vi "QueueDriver.vi"(0 "Queue Name":string, 5 "State":string, 7 "Array of States":string[](array[string]), 11 "error in (no error)":errorcluster, 13 "Operations":T1) -> (4 "Dequeued State":string, 15 "error out":errorcluster)   [LabVIEW 2020]
doc: "QueueDriver.vi is the SubVI which handles the states that is going to be operated in the Main VI."
uses:
  Typedefs/Operations.ctl
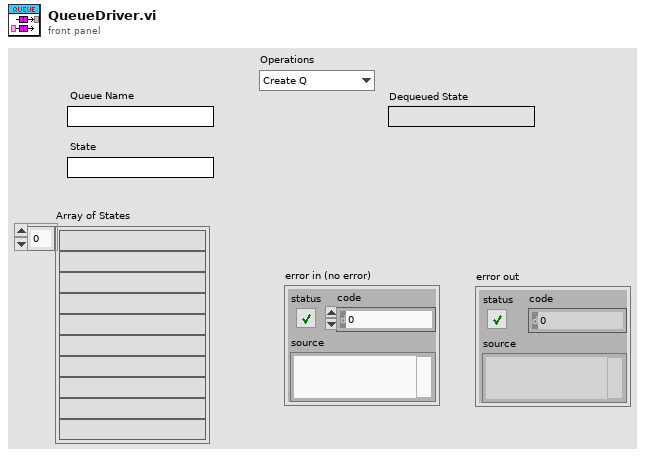
[diagram p1: front panel]
types:
  T1 = typedef "Operations.ctl" = enum16{"Create Q", "Enqueue 1", "Enqueue N", "Enstack 1", "Dequeue", "Flush Q", "Release Q"}
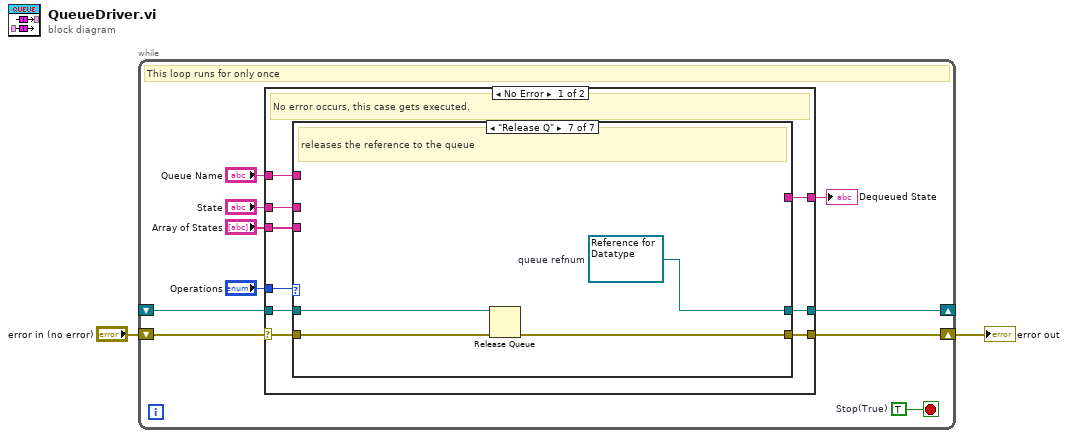
[diagram p0: block diagram]
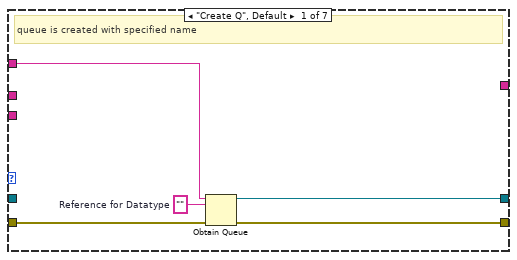
[diagram p2: hidden frame]
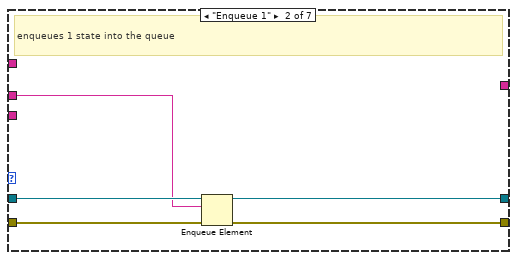
[diagram p3: hidden frame]
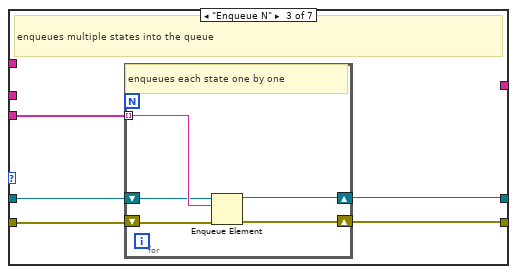
[diagram p4: hidden frame]
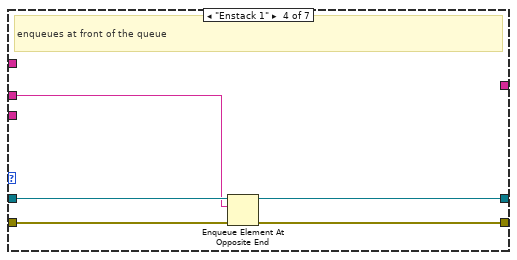
[diagram p5: hidden frame]
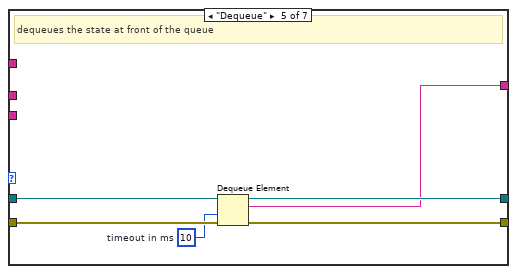
[diagram p6: hidden frame]
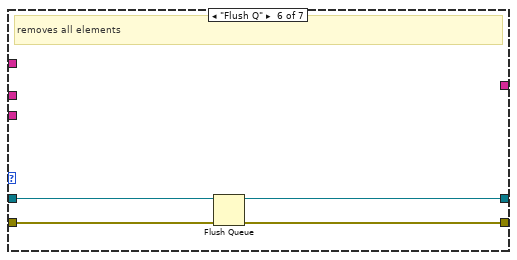
[diagram p7: hidden frame]
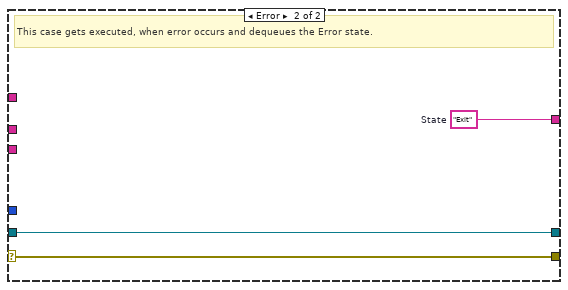
[diagram p8: hidden frame]
diagram:
  n1 = while {
    shift-right: [w10] -> w1
    shift-left: "error in (no error)" -> [w11]
    shift-right: [w8] -> _
    shift-left: _ -> [w7]
    stop <- w12 stop-if-true
    w12 = TRUE  # Stop(True)
    # "This loop runs for only once"
    n2 = case shown="No Error" w11 {
      selector: w11 -> [w21 w63]
      tunnel: [w20 w63] -> w10
      tunnel: [w17 w62] -> w9
      tunnel: [w19 w61] -> w8
      tunnel: w7 -> [w18 w61]
      tunnel: "Array of States" -> [w16 _]
      tunnel: "State" -> [w15 _]
      tunnel: "Queue Name" -> [w14 _]
      tunnel: "Operations" -> [w13 _]
      frame No Error {
        # "No error occurs, this case gets executed."
        n3 = case shown="\"Release Q\"" w13 {
          tunnel: w21 -> [w26 w31 w36 w46 w52 w56 w60]
          tunnel: [w25 w30 w35 w45 w51 w55 w59] -> w20
          tunnel: w14 -> [w24 _ _ _ _ _ _]
          tunnel: w15 -> [_ w27 _ w42 _ _ _]
          tunnel: w16 -> [_ _ w34 _ _ _ _]
          tunnel: [w22 w29 w33 w43 w48 w53 w57] -> w19
          tunnel: w18 -> [_ w28 w32 w44 w49 w54 w58]
          tunnel: [_ _ _ _ w47 _ _] -> w17
          frame "Create Q", Default {
            w23 = ""  # Reference for Datatype
            # "queue is created with specified name"
            n4 = Obtain Queue(name (unnamed)=w24, element data type=w23, error in (no error)=w26) -> (queue out=w22:refnum<queue>, error out=w25:errorcluster)  [unwired: 2 in, 1 out]
          }
          frame "Enqueue 1" {
            # "enqueues 1 state into the queue"
            n5 = Enqueue Element(queue=w28, element=w27, error in (no error)=w31) -> (queue out=w29:refnum<queue>, error out=w30:errorcluster)  [unwired: 1 in, 1 out]
          }
          frame "Enqueue N" {
            # "enqueues multiple states into the queue"
            n6 = for {
              shift-right: [w40] -> w35
              shift-left: w36 -> [w41]
              tunnel: w34 -> [w39] mode=indexing
              shift-right: [w38] -> w33
              shift-left: w32 -> [w37]
              # "enqueues each state one by one"
              n7 = Enqueue Element(queue=w37, element=w39, error in (no error)=w41) -> (queue out=w38:refnum<queue>, error out=w40:errorcluster)  [unwired: 1 in, 1 out]
            }
          }
          frame "Enstack 1" {
            # "enqueues at front of the queue"
            n8 = Enqueue Element At Opposite End(queue=w44, element=w42, error in (no error)=w46) -> (queue out=w43:refnum<queue>, error out=w45:errorcluster)  [unwired: 1 in, 1 out]
          }
          frame "Dequeue" {
            w50 = 10  # timeout in ms
            # "dequeues the state at front of the queue"
            n9 = Dequeue Element(queue=w49, timeout in ms (-1)=w50, error in (no error)=w52) -> (queue out=w48:refnum<queue>, element=w47:string, error out=w51:errorcluster)  [unwired: 1 out]
          }
          frame "Flush Q" {
            # "removes all elements"
            n10 = Flush Queue(queue=w54, error in (no error)=w56) -> (queue out=w53:refnum<queue>, error out=w55:errorcluster)  [unwired: 1 out]
          }
          frame "Release Q" {
            w57 = refnum<queue> refnum  # queue refnum
            # "releases the reference to the queue"
            n11 = Release Queue(queue=w58, error in (no error)=w60) -> (error out=w59:errorcluster)  [unwired: 1 in, 2 out]
          }
        }
      }
      frame Error {
        w62 = "Exit"  # State
        # "This case gets executed, when error occurs and dequeues the Error state."
      }
    }
    "Dequeued State" <- w9
  }
  "error out" <- w1
